vi "PH_BackreflectionMeas.Action Get data.vi"(0 "i ref in":refnum<vi>, 5 "error IO":errorcluster) -> (14 "i ref out":refnum<vi>, 19 "error out":errorcluster)   [LabVIEW 2014, in "PH_BackreflectionMeas.lvlib"]
doc: "This is the action within the proc case \"Get Data\": The data are analysied and indicated."
uses:
  PH_BackreflectionMeas.lvlib
  PH_TKTDS-30xx/PH_TKTDS-30xx.lvlib
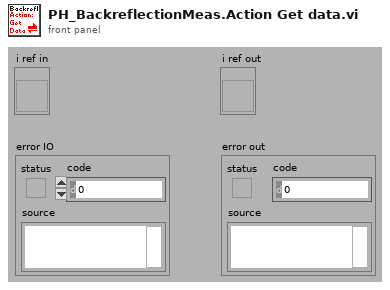
[diagram p1: front panel]
types:
  T1 = typedef "PH_BackreflectionMeas.lvlib/PH_BackreflectionMeas.i attribute.ctl" = cluster{"GUI Refs":cluster{"Get Data":refnum<vi>, "BR State":refnum<vi>, "Reset warning":refnum<vi>, "Low Energy Graph":refnum<vi>}, "Status":cluster{"Reset Warning":bool}, "Default Low Energy Chan Settings":T2, "Default High Energy Chan Settings":T2, "Default Trigger Settings":T3, "Default Acqu Settings":T4, "Limit [V]":dbl}
  T2 = typedef "PH_TKTDS-30xx.lvlib/PH_TKTDS-30xx.Channel Config.ctl" = cluster{"Channel Name":string, "Input Impedance":string, "Max Input Frequency":string, "Vertical Coupling":i32, "Channel Enabled":bool, "Probe Attenuation":dbl, "Vertical Range":dbl, "Vertical Offset":dbl}
  T3 = typedef "PH_TKTDS-30xx.lvlib/PH_TKTDS-30xx.Trigger Config.ctl" = cluster{"Source":string, "Slope":i32, "Level [V]":dbl}
  T4 = typedef "PH_TKTDS-30xx.lvlib/PH_TKTDS-30xx.Acquisition Config.ctl" = cluster{"Time base":dbl, "Record Length":u16, "Start Time":dbl, "Type":i32, "Continuous":bool}
  T5 = typedef "PH_TKTDS-30xx.lvlib/PH_TKTDS-30xx.i attribute.ctl" = cluster{"Default VISA Resource":string, "VISA Resource Name":refnum<visa-resource-name>, "Revision":cluster{"Instrument Driver":string, "Instrument Firmware":string}, "Selftest":cluster{"Result":u32, "Message":string}, "Channels":T2[], "Trigger Configuration":T3, "Acquisition Configuration":T4, "Fetched Waveforms":T6[], "GUI Refs":T7, "GUI Refs Channels":refnum<vi>[], "State":T8, "Error Message":string, "Allow Prdc Loop?":bool}
  T6 = typedef "PH_TKTDS-30xx.lvlib/PH_TKTDS-30xx.fetched Waveform.ctl" = cluster{"Source":string, "Actual Points":u32, "Initial X":dbl, "X Increment":dbl, "Waveform Array":dbl[]}
  T7 = typedef "PH_TKTDS-30xx.lvlib/PH_TKTDS-30xx.GUI Refs.ctl" = cluster{"Trigger":refnum<vi>, "Acquisition":refnum<vi>, "Graph":refnum<vi>, "State":refnum<vi>, "Delete":refnum<vi>, "Channel to be positioned":refnum<vi>, "Postion":refnum<vi>, "Display Intensity":refnum<vi>, "VISA Resource":refnum<vi>}
  T8 = typedef "PH_StatusHandler.lvlib/PH_StatusHandler.Status.ctl" = i16
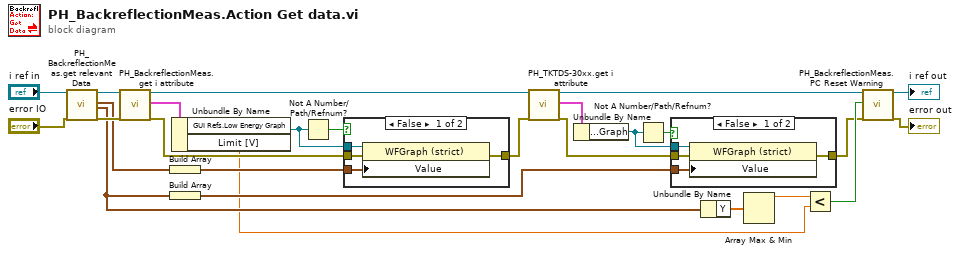
[diagram p0: block diagram]
diagram:
  n1 = call "PH_BackreflectionMeas.get relevant Data.vi"("i ref in"="i ref in", "error in"="error IO") -> ("i ref out"=w21:refnum<vi>, "low Energy Waveform"=w14:waveform(dbl), "high Energy Waveform"=w5:waveform(dbl), "error out"=w22:errorcluster)  [unwired: 14 in]
  n2 = call "PH_BackreflectionMeas.get i attribute.vi"("i ref in"=w21, "error in (no error)"=w22) -> ("i ref out"=w20:refnum<vi>, "i attribute"=w23:T1, "error out"=w19:errorcluster)  [unwired: 15 in]
  n3 = Build Array(w14) -> (w13:waveform(dbl)[])
  n4 = Build Array(w5) -> (w4:waveform(dbl)[])
  n5 = Unbundle By Name(w23) -> ("GUI Refs.Low Energy Graph"=w25:refnum<vi>, "Limit [V]"=w3:dbl)
  n6 = Not A Number/Path/Refnum?(number/path/refnum=w25) -> (NaN/Path/Refnum?=w18:bool)
  n7 = case shown="False" w18 {
    tunnel: w19 -> [w30 w31]
    tunnel: [w29 w31] -> w8
    tunnel: w25 -> [w28 _]
    tunnel: w13 -> [w27 _]
    frame False {
      n8 = property class="WFGraph (strict)"(reference=w28, error in=w30, "Value"=w27) -> (error out=w29:errorcluster)  [unwired: 1 out]
    }
    frame True {
    }
  }
  n9 = call "PH_TKTDS-30xx.get i attribute.vi"("i ref in"=w20, "error in (no error)"=w8) -> ("i ref out"=w10:refnum<vi>, "i attribute"=w7:T5, "error out"=w9:errorcluster)  [unwired: 15 in]
  n10 = Unbundle By Name(w7) -> ("GUI Refs.Graph"=w6:refnum<vi>)
  n11 = Not A Number/Path/Refnum?(number/path/refnum=w6) -> (NaN/Path/Refnum?=w11:bool)
  n12 = case shown="False" w11 {
    tunnel: w9 -> [w35 w36]
    tunnel: [w34 w36] -> w12
    tunnel: w6 -> [w33 _]
    tunnel: w4 -> [w32 _]
    frame False {
      n13 = property class="WFGraph (strict)"(reference=w33, error in=w35, "Value"=w32) -> (error out=w34:errorcluster)  [unwired: 1 out]
    }
    frame True {
    }
  }
  n14 = Unbundle By Name(w5) -> ("Y"=w15:dbl[])
  n15 = Array Max & Min(array=w15) -> (max value=w17:dbl)  [unwired: 3 out]
  n16 = Less?(x=w17, y=w3) -> (x < y?=w16:bool)
  n17 = call "PH_BackreflectionMeas.PC Reset Warning.vi"("i ref in"=w10, "Reset Warning?"=w16, "error in (no error)"=w12) -> ("i ref out"=→"i ref out":refnum<vi>, "error out"=→"error out":errorcluster)  [unwired: 15 in]
